vi "ZCAN_ReceiveData.vi"(3 "error in (no error)":errorcluster caption="错误输入（无错误）", 6 "can_handle":u32) -> (0 "error out":errorcluster caption="错误输出", 1 "Receive_Num":u32, 2 "ZCANDataObj（out）":T1[](array[typedef]))   [LabVIEW 2018]
doc: "该函数用于接收CAN报文。"
uses:
  data_type/ZCANDataObj.ctl
panel:
  in  "ZCANDataObj":T1
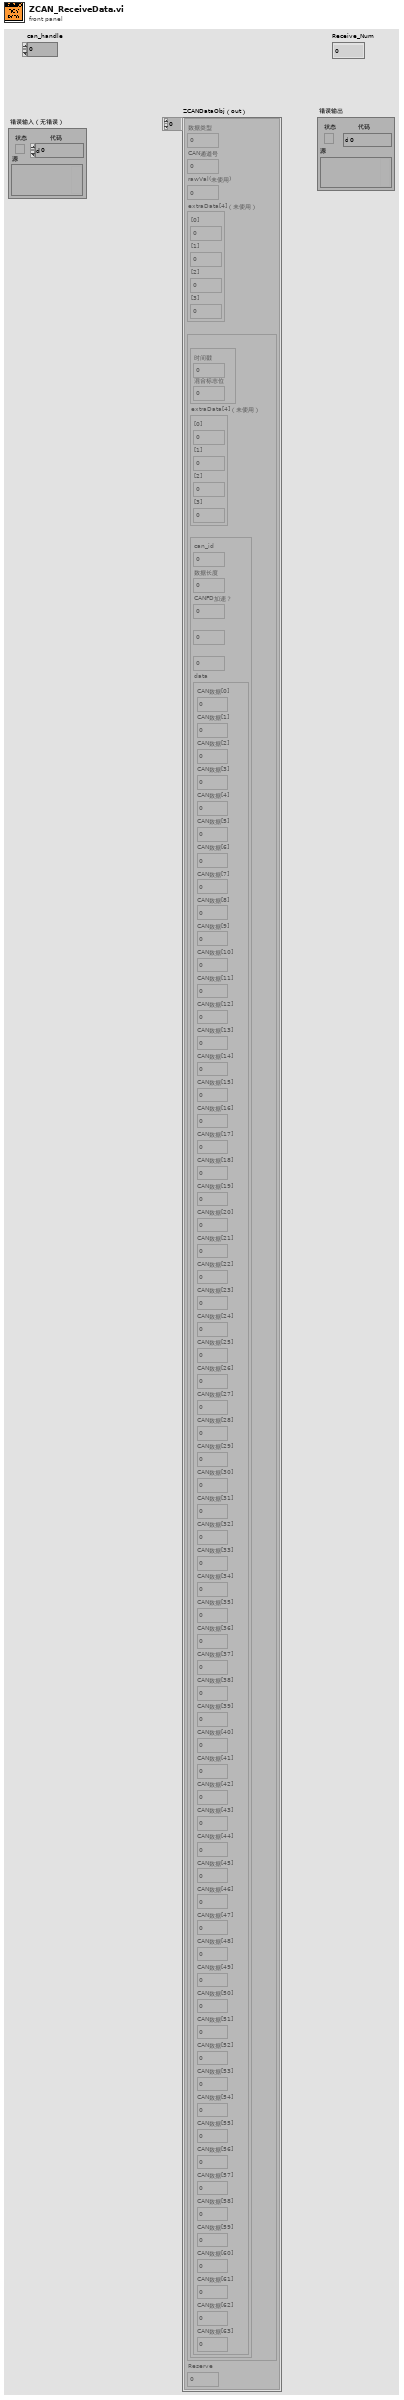
[diagram p1: front panel]
types:
  T1 = typedef "ZCANDataObj.ctl" = cluster{"数据类型":u8, "CAN通道号":u8, "rawVal(未使用)":u16, "extraData[4]（未使用）":cluster{"[0]":u8, "[1]":u8, "[2]":u8, "[3]":u8}, "canCANFDData":cluster{"时间戳+混合标志位":cluster{"时间戳":u64, "混合标志位":u32}, "extraData[4]（未使用）":cluster{"[0]":u8, "[1]":u8, "[2]":u8, "[3]":u8}, "frame":cluster{"can_id":u32, "数据长度":u8, "CANFD加速？":u8, "__res0":u8, "__res1":u8, "data":cluster{"CAN数据[0]":u8, "CAN数据[1]":u8, "CAN数据[2]":u8, "CAN数据[3]":u8, "CAN数据[4]":u8, "CAN数据[5]":u8, "CAN数据[6]":u8, "CAN数据[7]":u8, "CAN数据[8]":u8, "CAN数据[9]":u8, "CAN数据[10]":u8, "CAN数据[11] ":u8, "CAN数据[12] ":u8, "CAN数据[13] ":u8, "CAN数据[14] ":u8, "CAN数据[15] ":u8, "CAN数据[16]":u8, "CAN数据[17]":u8, "CAN数据[18]":u8, "CAN数据[19]":u8, "CAN数据[20]":u8, "CAN数据[21]":u8, "CAN数据[22]":u8, "CAN数据[23]":u8, "CAN数据[24] ":u8, "CAN数据[25]":u8, "CAN数据[26]":u8, "CAN数据[27]":u8, "CAN数据[28]":u8, "CAN数据[29]":u8, "CAN数据[30]":u8, "CAN数据[31]":u8, "CAN数据[32]":u8, "CAN数据[33]":u8, "CAN数据[34]":u8, "CAN数据[35]":u8, "CAN数据[36]":u8, "CAN数据[37]":u8, "CAN数据[38]":u8, "CAN数据[39]":u8, "CAN数据[40]":u8, "CAN数据[41]":u8, "CAN数据[42]":u8, "CAN数据[43]":u8, "CAN数据[44]":u8, "CAN数据[45]":u8, "CAN数据[46]":u8, "CAN数据[47]":u8, "CAN数据[48]":u8, "CAN数据[49]":u8, "CAN数据[50]":u8, "CAN数据[51]":u8, "CAN数据[52]":u8, "CAN数据[53]":u8, "CAN数据[54]":u8, "CAN数据[55]":u8, "CAN数据[56]":u8, "CAN数据[57]":u8, "CAN数据[58]":u8, "CAN数据[59]":u8, "CAN数据[60]":u8, "CAN数据[61]":u8, "CAN数据[62]":u8, "CAN数据[63]":u8}}}, "Reserve":u32}
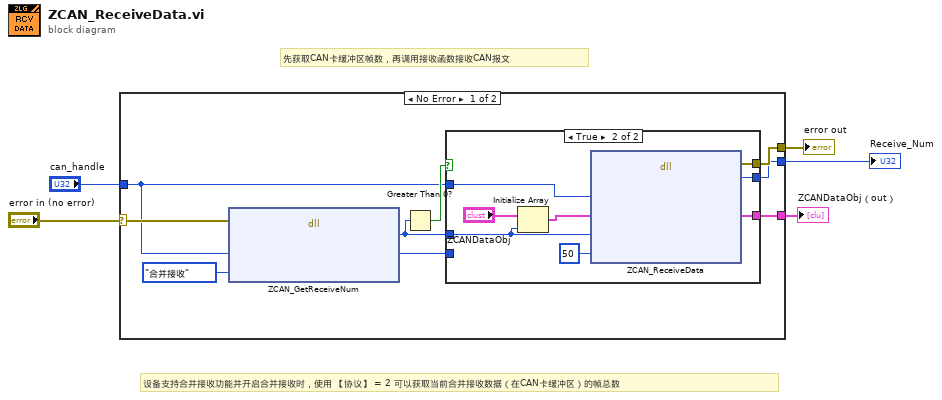
[diagram p0: block diagram]
diagram:
  # "先获取CAN卡缓冲区帧数，再调用接收函数接收CAN报文"
  # "设备支持合并接收功能并开启合并接收时，使用 【协议】 = 2 可以获取当前合并接收数据（在CAN卡缓冲区）的帧总数"
  n1 = case shown="No Error" "error in (no error)" {
    selector: "error in (no error)" -> [w14 _]
    tunnel: "can_handle" -> [w9 _]
    tunnel: [w7 _] -> w3
    tunnel: [w10 _] -> w1
    tunnel: [w8 _] -> w2
    frame No Error {
      n2 = dll-call lib="PTH2qabs CUsersadminDesktopzlgcan_demo_20220516_2018版本zlgcan_demo_USBCANFD_mergebinzlgcan_wrap.dll" fn="ZCAN_GetReceiveNum"(error in=w14, "通道句柄"=w9, "协议"=enum16{"CAN", "CANFD", "合并接收"}."合并接收") -> ("缓冲区帧数"=w11:u32, "通道句柄"=w12:u32)  [unwired: 3 in, 2 out]
      n3 = Greater Than 0?(x=w11) -> (x > 0?=w13:bool)
      n4 = case shown="True" w13 {
        tunnel: w12 -> [_ _]
        tunnel: w11 -> [_ w16]
        tunnel: [_ w21] -> w10
        tunnel: [_ w20] -> w8
        tunnel: [_ w19] -> w7
        tunnel: w9 -> [_ w18]
        frame False {
        }
        frame True {
          n5 = Initialize Array("ZCANDataObj", w16) -> (w15:T1[])
          n6 = dll-call lib="PTH2qabs CUsersadminDesktopzlgcan_demo_20220516_2018版本zlgcan_demo_USBCANFD_mergebinzlgcan_wrap.dll" fn="ZCAN_ReceiveData"("通道句柄"=w18, "数据帧数组"=w15, "数据帧数"=w16, "超时时间"=50) -> (error out=w20:errorcluster, "已接收帧数"=w19:u32, "数据帧数组"=w21:T1[])  [unwired: 6 in, 1 out]
        }
      }
    }
    frame Error {
    }
  }
  "Receive_Num" <- w3
  "error out" <- w2
  "ZCANDataObj（out）" <- w1
